vi "Global_내구.vi"() -> ()   [LabVIEW 2019]
panel:
  in  "manual?":bool
  out "dup path":path
  in  "Waveform_DL950":refnum<vi>
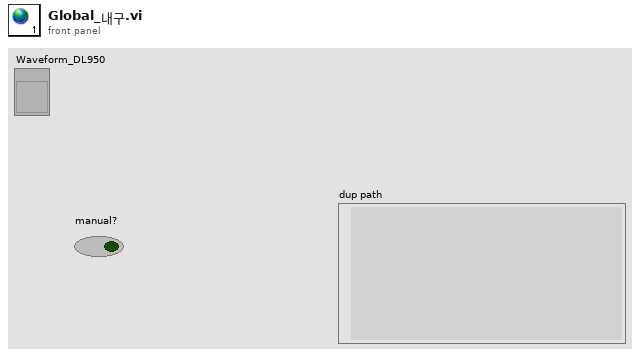
[diagram p1: front panel]
diagram:
